vi "servo_subvi.vi"(6 "Turns":bool, 7 "error in (no error)":errorcluster, 8 "LINX Resource":T1, 9 "Servo Channel":u8, 10 "Speed":u32) -> (0 "error out":errorcluster, 2 "Position":dbl, 3 "LINX Resource out":T1)   [LabVIEW 2020]
uses:
  <vilib>/MakerHub/LINX/Private/Type Defs/LINX Ref.ctl
  <vilib>/MakerHub/LINX/Private/Type Defs/Platform.ctl
  <vilib>/MakerHub/LINX/Private/Type Defs/Interface.ctl
  <vilib>/MakerHub/LINX/Private/Device/Type Defs/LINX Device Config.ctl
  <vilib>/MakerHub/LINX/Private/Device/Type Defs/TCP Config.ctl
  <vilib>/MakerHub/LINX/Private/Device/Type Defs/Channels.ctl
  <vilib>/MakerHub/LINX/Public/Sensors/Motion/Servo/Servo Set Pulse Width One Channel.vi
  <vilib>/MakerHub/LINX/Public/Sensors/Motion/Servo/Servo.lvlib
  <vilib>/Analysis/NI_AALPro.lvlib
  <vilib>/MakerHub/LINX/LMH-LINX.lvlib
  <vilib>/MakerHub/LINX/Private/Device/Device.lvlib
panel:
  out "Position out":dbl
  in  "Position in":dbl format="%0.2f"
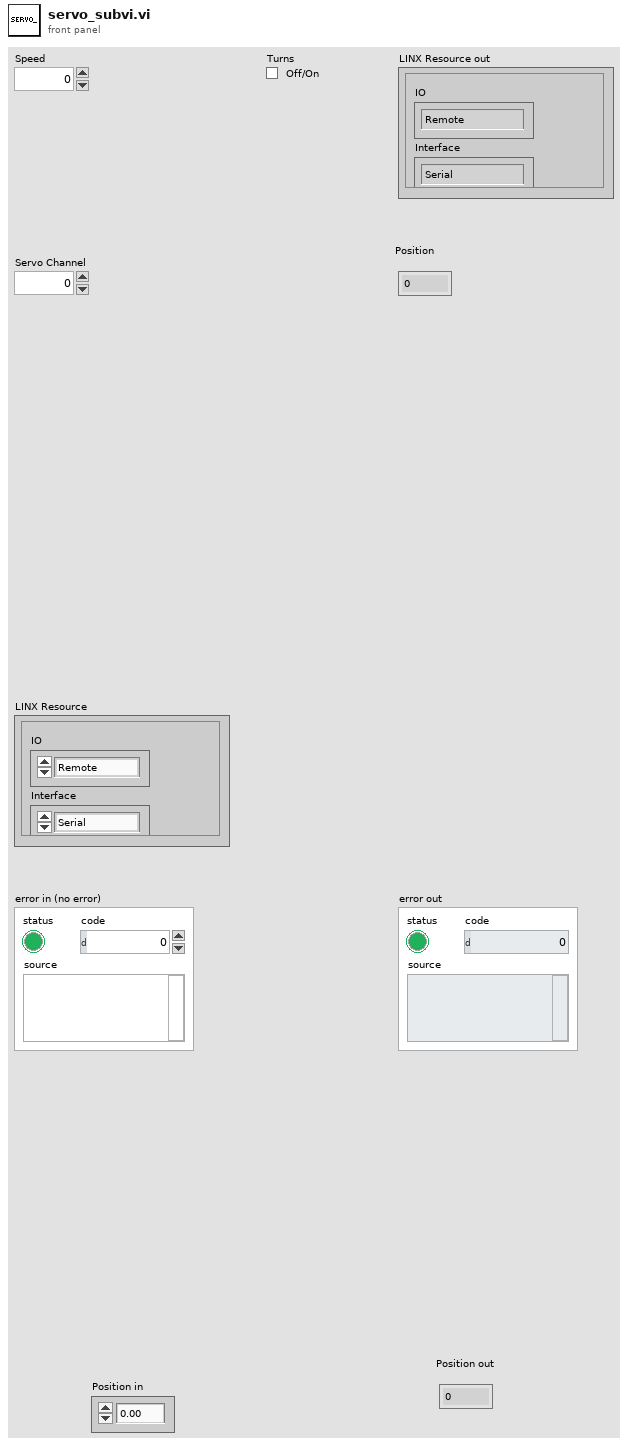
[diagram p1: front panel]
types:
  T1 = typedef "LMH-LINX.lvlib/LINX Ref.ctl" = cluster{"IO":T2, "Interface":T3, "LINX Device Config":T4}
  T2 = typedef "LMH-LINX.lvlib/Platform.ctl" = enum16{"Remote", "Local"}
  T3 = typedef "LMH-LINX.lvlib/Interface.ctl" = enum16{"Serial", "TCP"}
  T4 = typedef "LMH-LINX.lvlib/Device.lvlib/LINX Device Config.ctl" = cluster{"Interface":T3, "COM Port":refnum<visa-resource-name>, "TCP Configuration":T5, "Device Family":u8, "Device ID":u8, "Device Name":string, "TCP Ref":refnum<k5>, "Channels":T6}
  T5 = typedef "LMH-LINX.lvlib/Device.lvlib/TCP Config.ctl" = cluster{"IP Address":string, "Port":u16}
  T6 = typedef "LMH-LINX.lvlib/Channels.ctl" = cluster{"DI":u8[], "DO":u8[], "AI":u8[], "AO":u8[], "PWM":u8[], "QE":u8[], "UART":u8[], "I2C 2":u8[], "SPI":u8[], "CAN":u8[], "Servo":u8[], "AI Ref (V)":dbl, "AI Resolution (Bits)":u8, "AO Ref (V)":dbl, "AO Resolution (Bits)":u8}
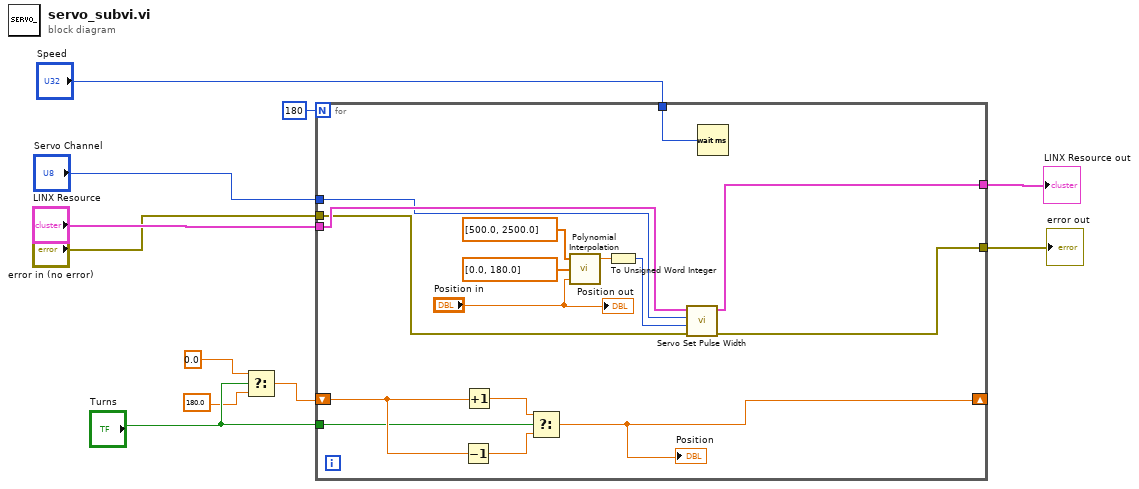
[diagram p0: block diagram]
diagram:
  n1 = Select(t=0.0, s="Turns", f=180.0) -> (s? t:f=w3:dbl)
  n2 = for {
    N: 180 -> [_]
    tunnel: "error in (no error)" -> [w15]
    tunnel: "Servo Channel" -> [w14]
    tunnel: "LINX Resource" -> [w16]
    tunnel: "Speed" -> [w27]
    shift-right: [w22] -> _
    shift-left: w3 -> [w26]
    tunnel: "Turns" -> [w23]
    tunnel: [w13] -> w2
    tunnel: [w12] -> w1
    n3 = Decrement(x=w26) -> (x-1=w24:dbl)
    n4 = Increment(x=w26) -> (x+1=w25:dbl)
    n5 = Select(t=w25, s=w23, f=w24) -> (s? t:f=w22:dbl)
    "Position" <- w22
    n6 = call <vilib>:"Polynomial Interpolation.vi"("x value"="Position in", "X"=dbl[] [0.0, 180.0], "Y"=dbl[] [500.0, 2500.0]) -> ("interpolation value"=w21:dbl)  [unwired: 2 out]
    n7 = To Unsigned Word Integer(number=w21) -> (unsigned 16bit integer=w20:u16)
    n8 = call-poly <vilib>:"Servo Set Pulse Width.vi"("Error In"=w15, "Pulse Width (uS)"=w20, "Servo Channel"=w14, "LINX Resource"=w16) -> ("Error Out"=w12:errorcluster, "LINX Resource"=w13:T1)  [unwired: 6 in]
    n9 = Wait (ms)(milliseconds to wait=w27) -> ()  [unwired: 1 out]
    "Position out" <- "Position in"
  }
  "LINX Resource out" <- w2
  "error out" <- w1
